vi "FPGA Main Default.vi"() -> ()   [LabVIEW 2016]
doc: "The myRIO v1.1 FPGA Shipping Personality. This personality contains support for:\n- 2 Analog Input Interrupt channel\n- 4 Digital Input Interrupt channel\n- 1 Timer\n- 1 Accelerometer\n- 1 Button\n- 4 LED\n- 10 Analog Input channels with 1 Sample\n- 6 Analog Output channels with 1 Sample\n- 40 Digital I/O channels with 1 Sample\n- 2 I2C channels\n- 4 Encoder channels\n- 6 PWM channels\n- 2 SPI channels"
uses:
  Sub VIs/Utilities/Start Boolean.ctl
  <vilib>/Platform/TimedLoop/XDataNode/timing_clust.ctl
  <vilib>/Platform/TimedLoop/XDataNode/nitl_modes.ctl
  <vilib>/Platform/TimedLoop/XDataNode/wakeup.ctl
  <vilib>/rvi/Emulation/niFpgaGetClockAttributes.vi
  <vilib>/rvi/Emulation/niFpgaSctlEmulationGetInTimedLoop.vi
  <vilib>/rvi/Emulation/niFpgaEmulationReportErrorSimple.vi
  <vilib>/rvi/eio/common/nirviEmuTemplateMethod_errors.vi
  <vilib>/rvi/Emulation/niFpgaCriticalErrorInLSC.vi
  <vilib>/rvi/Emulation/niFpgaProcessEmulError.vi
  <vilib>/rvi/Emulation/niFpgaEmulationIsFPGAContextNoSignature.vi
  <vilib>/rvi/errors/niFpgaSetErrorForExecOnDevCompSimple.vi
  <vilib>/rvi/eio/common/nirviEmuReportErrorAndStop.vi
  <vilib>/rvi/DataTransferAndStorage/Container/Common/niFpgaContainerGetUniqueNameForEmu.vi
  <vilib>/rvi/FIFO/Fifo_Resource/nirvififoEmulationSetSize.vi
  <vilib>/rvi/FIFO/Fifo_Resource/nirviFifoEmulationQueueMgr.vi
  <instcachedir>/0/nirviFifoEmulationQueueMgr_E5CAEC123FF24DC58D834DCA3CDAA9B5.lvgen/nirviFifoEmulationQueueMgr_E5CAEC123FF24DC58D834DCA3CDAA9B5_002.vi
  <vilib>/rvi/FIFO/Fifo_Resource/nirvififoEmulationDetermineInputValidOut.vi
  <vilib>/rvi/FIFO/Fifo_Resource/nirvififoEmulationCreateLock.vi
  <vilib>/rvi/FIFO/Fifo_Resource/nirvififoEmulationObtainLock.vi
  <vilib>/rvi/FIFO/Fifo_Resource/nirvififoEmulationReleaseLock.vi
  <vilib>/rvi/occurrence/nirviWaitOnOccurrenceBase.vi
  <vilib>/rvi/errors/nirviReportUnexpectedCaseInternalError.vi
  <vilib>/rvi/errors/nirviReportUnexpectedCaseInternalError (U32).vi
  <vilib>/Utility/error.llb/Clear Errors.vi
  <vilib>/rvi/DataTransferAndStorage/Container/Common/niFpgaContainerSetEmuInfo.vi
  <vilib>/eio/EIONode/EIONode.xnode
  <vilib>/rvi/DataTransferAndStorage/Container/XNode/niFpgaContainer.xnode
  <vilib>/rvi/FIFO/Fifo_Resource/nirvififoEmulationWrite.vi
  <vilib>/rvi/FIFO/Fifo_Resource/nirvififoEmulationRead.vi
  <vilib>/Platform/TimedLoop/XDataNode/XDataNode.xnode
  <vilib>/rvi/LocalResourceManager/LocalResourceManager.xnode
  <vilib>/Platform/TimedLoop/XDataNode/XDNodeRunTimeDep.lvlib
panel:
  in  "AO.A_0.VAL":u16
  in  "AO.A_1.VAL":u16
  in  "AO.B_0.VAL":u16
  in  "AO.B_1.VAL":u16
  out "AI.B_3.VAL":u16
  out "AI.B_2.VAL":u16
  out "AI.B_1.VAL":u16
  out "AI.B_0.VAL":u16
  out "AI.A_3.VAL":u16
  out "AI.A_2.VAL":u16
  out "AI.A_1.VAL":u16
  out "AI.A_0.VAL":u16
  out "DIO.B_7:0.IN":u8 format="%08b"
  in  "DIO.B_7:0.DIR":u8 format="%08b"
  in  "DIO.B_7:0.OUT":u8 format="%08b"
  in  "PWM.A_2.CS":u8=1
  in  "PWM.A_2.CNFG":u8=4
  out "PWM.A_2.CNTR":u16
  in  "PWM.A_2.MAX":u16=39999
  in  "PWM.A_2.CMP":u16=20000
  in  "PWM.A_1.CS":u8=1
  in  "PWM.A_1.CNFG":u8=4
  out "PWM.A_1.CNTR":u16
  in  "PWM.A_1.MAX":u16=39999
  in  "PWM.A_1.CMP":u16=20000
  in  "PWM.A_0.CS":u8=1
  in  "PWM.A_0.CNFG":u8=4
  out "PWM.A_0.CNTR":u16
  in  "PWM.A_0.CMP":u16=20000
  in  "PWM.A_0.MAX":u16=39999
  in  "SPI.A.DATO":u16
  out "SPI.A.DATI":u16
  in  "SPI.A.CNFG":u16=112
  in  "SPI.A.CNT":u16=19
  in  "SPI.B.CNT":u16=19
  in  "SPI.B.CNFG":u16=112 format="%0.0f"
  out "SPI.B.DATI":u16
  in  "SPI.B.DATO":u16
  in  "ENC.A.CNFG":u8 format="%08b"
  in  "ENC.B.CNFG":u8 format="%08b"
  out "ENC.A.CNTR":u32
  out "ENC.B.CNTR":u32
  out "ENC.A.STAT":u8 format="%08b"
  out "ENC.B.STAT":u8 format="%08b"
  in  "SPI.A.GO":T1
  out "SPI.A.STAT":u8 format="%08b"
  in  "SPI.B.GO":T1
  out "SPI.B.STAT":u8 format="%08b"
  out "I2C.B.STAT":u8 format="%08b"
  in  "I2C.B.CNTL":u8 format="%08b"
  out "I2C.A.STAT":u8 format="%08b"
  in  "I2C.A.CNTL":u8 format="%08b"
  in  "I2C.B.CNTR":u8=213
  in  "I2C.B.ADDR":u8 format="%08.0f"
  out "I2C.B.DATI":u8
  in  "I2C.B.DATO":u8
  in  "I2C.A.CNTR":u8=213
  in  "I2C.A.ADDR":u8 format="%08b"
  out "I2C.A.DATI":u8
  in  "I2C.A.DATO":u8
  in  "I2C.B.CNFG":u8=1 format="%08b"
  in  "I2C.A.CNFG":u8=1 format="%08b"
  in  "I2C.A.GO":T1
  in  "I2C.B.GO":T1
  out "SYS.AI.RDY":bool
  out "SYS.RDY":bool
  in  "PWM.B_2.CS":u8=1
  in  "PWM.B_2.CNFG":u8=4
  out "PWM.B_2.CNTR":u16
  in  "PWM.B_2.MAX":u16=39999
  in  "PWM.B_2.CMP":u16=20000
  in  "PWM.B_1.CS":u8=1
  in  "PWM.B_1.CNFG":u8=4
  out "PWM.B_1.CNTR":u16
  in  "PWM.B_1.MAX":u16=39999
  in  "PWM.B_1.CMP":u16=20000
  in  "PWM.B_0.CS":u8=1
  in  "PWM.B_0.CNFG":u8=4
  out "PWM.B_0.CNTR":u16
  in  "PWM.B_0.MAX":u16=39999
  in  "PWM.B_0.CMP":u16=20000
  out "DIO.A_7:0.IN":u8 format="%08b"
  in  "DIO.A_7:0.OUT":u8 format="%08b"
  in  "DIO.A_7:0.DIR":u8 format="%08b"
  out "AI.C_1.VAL":u16
  out "AI.C_0.VAL":u16
  in  "AO.C_0.VAL":u16
  in  "AO.C_1.VAL":u16
  in  "SYS.SELECTB":u8 format="%08b"
  in  "SYS.SELECTA":u8 format="%08b"
  out "DIO.A_15:8.IN":u8 format="%08b"
  in  "DIO.A_15:8.OUT":u8 format="%08b"
  in  "DIO.A_15:8.DIR":u8 format="%08b"
  out "DIO.B_15:8.IN":u8 format="%08b"
  in  "DIO.B_15:8.DIR":u8 format="%08b"
  in  "DIO.B_15:8.OUT":u8 format="%08b"
  out "AI.AudioIn_R.VAL":u16
  out "AI.AudioIn_L.VAL":u16
  in  "AO.AudioOut_R.VAL":u16
  in  "AO.AudioOut_L.VAL":u16
  in  "AO.SYS.GO":T1
  out "ACC.X.VAL":u16
  out "ACC.Y.VAL":u16
  out "SYS.ACC.RDY":bool
  out "ACC.Z.VAL":u16
  in  "DO.LED3:0":u8 format="%04b"
  out "DI.BTN":u8 format="%08b"
  out "AO.SYS.STAT":bool
  in  "IRQ.AI_A_3:0.CNFG":u8 format="%.0b"
  in  "IRQ.AI_A_0.THRESHOLD":u16
  in  "IRQ.AI_A_1.THRESHOLD":u16
  in  "IRQ.AI_A_0.NO":u8
  in  "IRQ.AI_A_1.NO":u8
  in  "IRQ.DIO_A_7:0.ENA":u8 format="%08b"
  in  "IRQ.DIO_A_7:0.RISE":u8 format="%08b"
  in  "IRQ.DIO_A_7:0.FALL":u8 format="%08b"
  in  "IRQ.DIO_A_0.NO":u8
  in  "IRQ.DIO_A_1.NO":u8
  in  "IRQ.DIO_A_2.NO":u8
  in  "IRQ.DIO_A_3.NO":u8
  in  "IRQ.DIO_A_3.CNT":u32
  in  "IRQ.DIO_A_2.CNT":u32
  in  "IRQ.DIO_A_1.CNT":u32
  in  "IRQ.DIO_A_0.CNT":u32
  in  "IRQ.AI_A_1.HYSTERESIS":u16=17
  in  "IRQ.TIMER.WRITE":u32
  in  "IRQ.TIMER.SETTIME":T1
  out "IRQ.TIMER.READ":u32
  in  "SPI.A.IRQ.NO":u8=15
  in  "SPI.B.IRQ.NO":u8=15
  in  "IRQ.AI_A_0.HYSTERESIS":u16=17
  in  "IRQ.DI_BTN.ENA":bool
  in  "IRQ.DI_BTN.RISE":bool
  in  "IRQ.DI_BTN.FALL":bool
  in  "IRQ.DI_BTN.CNT":u32
  in  "IRQ.DI_BTN.NO":u8
  # "System"
  # "Onboard Devices"
  # "Connector A"
  # "Connector B"
  # "Connector C"
  # "Audio Connector"
  # "Accelerometer"
  # "Analog Input"
  # "Analog Output"
  # "Digital I/O"
  # "PWM"
  # "SPI Master"
  # "Analog Input"
  # "Analog Output"
  # "Digital I/O"
  # "PWM"
  # "SPI Master"
  # "Analog Input"
  # "Analog Output"
  # "Digital I/O"
  # "Counters / PWM"
  # "Analog Input"
  # "Analog Output"
  # "IO Configuration"
  # "IO Configuration"
  # "IO Configuration"
  # "Encoders"
  # "Buttons & LEDs"
  # "Analog Interrupt"
  # "Digital Interrupt"
  # "Encoders"
  # "Encoders"
  # "Button Interrupt"
  # "I2C Master"
  # "I2C Master"
  # "Timer Interrupt"
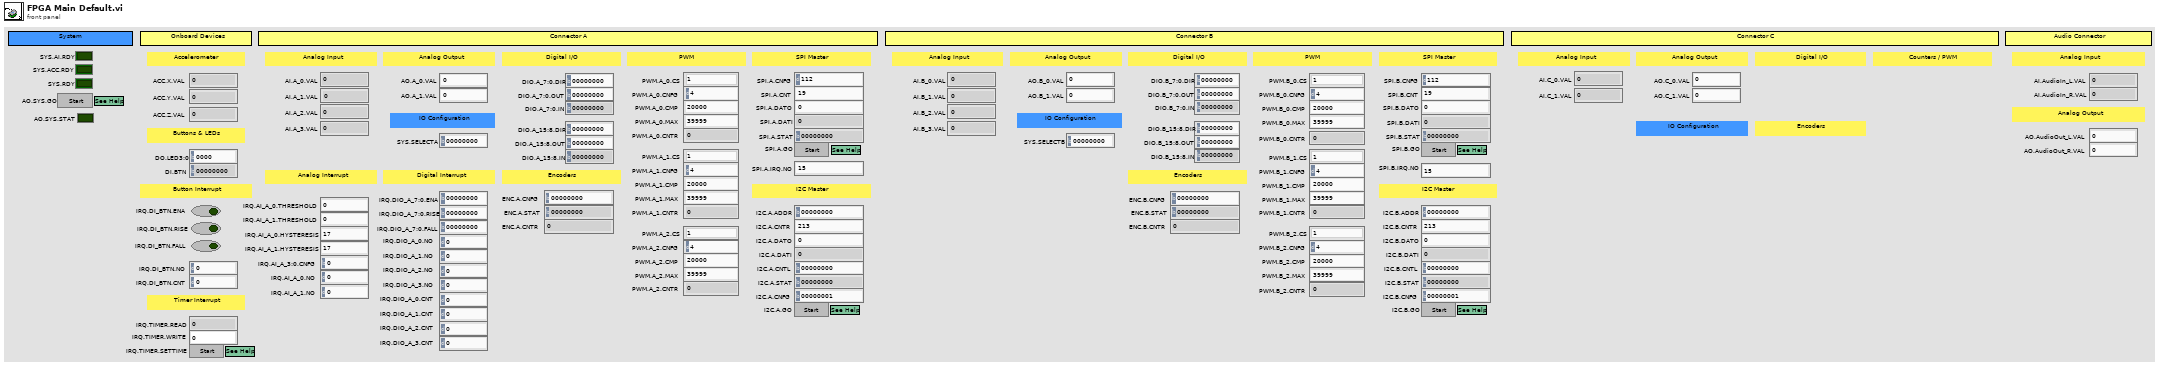
[diagram p1: front panel]
types:
  T1 = typedef "Start Boolean.ctl" = bool
  T2 = typedef "XDNodeRunTimeDep.lvlib/timing_clust.ctl" = cluster{"Expected End [f-1]":u64, "Actual End [f-1]":u64, "Finished Late? [f-1]":bool, "Expected End [i-1]":u64, "Actual End [i-1]":u64, "Finished Late? [i-1]":bool, "Expected Start [i]":u64, "Actual Start [i]":u64, "Expected Start [f]":u64, "Actual Start [f]":u64, "Source Name":string, "Structure Name":string, "Period":i64, "Deadline":i64, "Offset":i64, "Start":i64, "Priority":i32, "Timeout":i32, "Mode":T3, "Wakeup Reason":T4, "Error":errorcluster, "Source Type":string, "Secondary Source Type":string, "Global End Time":u64, "Global Start Time":u64, "Frame Duration":u64, "Iteration Duration":u64, "Assigned CPU":i32, "I/O Scan Engine Mode":u32}
  T3 = typedef "XDNodeRunTimeDep.lvlib/nitl_modes.ctl" = enum32{"No Change", "Process missed periods, maintain original phase", "Discard missed periods, maintain original phase", "Process missed periods, ignore original phase", "Discard missed periods, ignore original phase"}
  T4 = typedef "XDNodeRunTimeDep.lvlib/wakeup.ctl" = enum32{"Normal", "Aborted", "Asynchronous wakeup", "Timing source error", "Timed loop error", "Timeout"}
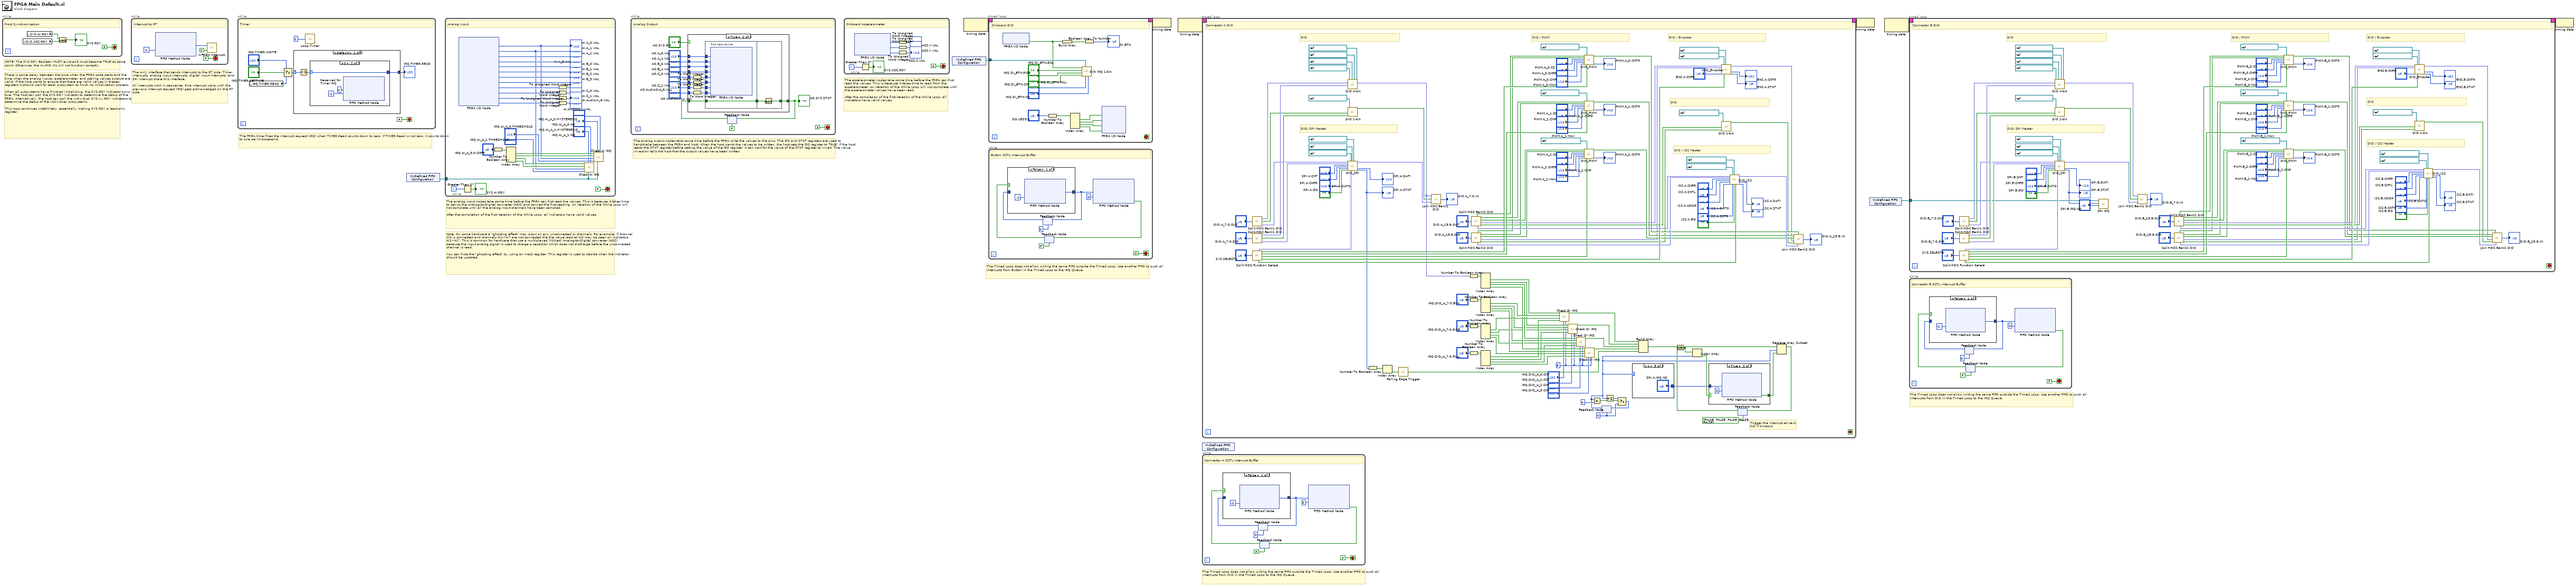
[diagram p0: block diagram]
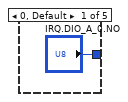
[diagram p9: hidden frame]
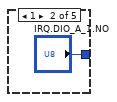
[diagram p10: hidden frame]
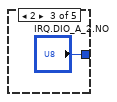
[diagram p11: hidden frame]
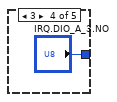
[diagram p12: hidden frame]
diagram:
  # "The Timed Loop does not allow writing the same FIFO outside the Timed Loop. Use another FIFO to push all interrupts from DIO in the Timed Loop to the IRQ Queue."
  # "The Timed Loop does not allow writing the same FIFO outside the Timed Loop. Use another FIFO to push all interrupts from Button in the Timed Loop to the IRQ Queue."
  # "The Timed Loop does not allow writing the same FIFO outside the Timed Loop. Use another FIFO to push all interrupts from DIO in the Timed Loop to the IRQ Queue."
  # "The accelerometer nodes take some time before the FPGA can first read the values. This is because it takes time to read from the accelerometer. An iteration of the While Loop will not complete until the accelerometer values have been read.\n\nAfter the completion of the first iteration of the While Loop, all indicators have valid values."
  # "The analog output nodes take some time before the FPGA write the values to the pins. The GO and STAT registers are used to handshake between the FPGA and host. When the host wants the values to be written, the host sets the GO register to TRUE. If the host reads the STAT register before setting the value of the GO register, it can wait for the value of the STAT register to invert. The value inversion tells the host that the output values have been written."
  # "The analog input nodes take some time before the FPGA can first read the values. This is because it takes time to set up the Analog-to-Digital converter (ADC) and convert the first reading. An iteration of the While Loop will not complete until all the analog input channels have been sampled.\n\nAfter the completion of the first iteration of the While Loop, all indicators have valid values."
  # "Note: On some hardware a \"ghosting effect\" may occur on any unconnected AI channels. For example, if channel AI0 is connected and channels AI1~AI7 are not connected the the value read at AI0 may be seen on indicators AI1~AI7. This is common for hardware that use a multiplexed (MUXed) Analog-to-Digital converter (ADC), because the input analog signal is used to charge a capacitor which does not discharge before the unconnected channel is read.\n\nYou can hide the \"ghosting effect\" by using an mask register. This register is used to decide when the indicator should be updated."
  # "The FPGA timer fires the interrupt request (IRQ) when TIMER.Read counts down to zero. If TIMER.Read is not zero, it counts down to one per microsecond."
  # "The only interface that sends interrupts to the RT side. Timer interrupts, analog input interrupts, digital input interrupts, and SPI interrupt share this interface.\n\nAll interrupts work in sequence. One interrupt waits until the previous interrupt request (IRQ) gets acknowledged on the RT side."
  # "NOTE: The SYS.RDY Boolean MUST exist and must become TRUE at some point. Otherwise, the myRIO VIs will not function correctly."
  # "There is some delay between the time when the FPGA code starts and the time when the analog inputs, accelerometer, and scaling values outputs are valid. If the host wants to ensure that there are valid values in theses registers it should wait for each subsystem to finish its initialization process. \n\nWhen all subsystems have finished initializinig, the SYS.RDY indicator turns true. The host can poll the SYS.RDY indicator to determine the status of the FPGA. Alternatively, the host can poll the individual SYS.xx.RDY indicators to determine the status of the individual subsystems.\n\nThis loop continues indefinitely, essentially making SYS.RDY a read-only register."
  n1 = while {
    stop <- FALSE stop-if-true
    # "Host Synchronization"
    n2 = local read "SYS.ACC.RDY"() -> (w11:bool)
    n3 = local read "SYS.AI.RDY"() -> (w13:bool)
    n4 = Compound Arithmetic op=AND(w13, w11) -> (→"SYS.RDY":bool)
  }
  n5 = while {
    stop <- FALSE stop-if-true
    # "Interrupt to RT"
    n6 = xnode ("FIFO Method Node")("Timeout"=-1) -> ("Element"=w16:u8)  [unwired: 1 in, 2 out]
    n7 = call <vilib>:"niFPGA Interrupt.vi"("Wait Until Cleared (F)"=TRUE, "IRQ Number (0)"=w16) -> ()  [unwired: 1 in]
  }
  n8 = while {
    stop <- FALSE stop-if-true
    # "Timer"
    n9 = local read "IRQ.TIMER.READ"() -> (w21:u32)
    n10 = Select(t="IRQ.TIMER.WRITE", s="IRQ.TIMER.SETTIME", f=w21) -> (s? t:f=w19:u32)
    n11 = case shown="Default" w19 {
      selector: w19 -> [w25 w28]
      tunnel: [w25 w26] -> w18
      frame 0 {
      }
      frame Default {
        n12 = Decrement(x=w28) -> (x-1=w27:u32)
        n13 = case shown="0" w27 {
          selector: w27 -> [w29 w32]
          tunnel: [w29 w32] -> w26
          frame Default {
          }
          frame 0 {
            w31 = u8 0  # Reserved for Timer IRQ
            n14 = xnode ("FIFO Method Node")("Element"=w31, "Timeout"=-1) -> ()  [unwired: 1 in, 2 out]
          }
        }
      }
    }
    "IRQ.TIMER.READ" <- w18
    n15 = call "Loop Timer"("Count(uSec)"=u8 1 ("Count(mSec)")) -> ()  [unwired: 1 out]
  }
  n16 = xnode "VI-Defined FIFO Configuration"() -> ("FIFO Out"=w3:refnum<k21>)
  n17 = while {
    tunnel: w3 -> [w34]
    i -> [w61]
    stop <- FALSE stop-if-true
    # "Analog Input"
    n18 = xnode "FPGA I/O Node"() -> ("ConnectorA/AI0"=w39:u16, "ConnectorA/AI1"=w38:u16, "ConnectorA/AI2"=→"AI.A_2.VAL":u16, "ConnectorA/AI3"=→"AI.A_3.VAL":u16, "ConnectorB/AI0"=→"AI.B_0.VAL":u16, "ConnectorB/AI1"=→"AI.B_1.VAL":u16, "ConnectorB/AI2"=→"AI.B_2.VAL":u16, "ConnectorB/AI3"=→"AI.B_3.VAL":u16, "ConnectorC/AI0"=w55:i16, "ConnectorC/AI1"=w54:i16, "AudioIn/Left"=w53:i16, "AudioIn/Right"=w52:i16)  [unwired: 12 in, 12 out]
    "AI.A_0.VAL" <- w39
    "AI.A_1.VAL" <- w38
    n19 = Greater Than 0?(x=w61) -> (x > 0?=→"SYS.AI.RDY":bool)
    n20 = Number To Boolean Array(number="IRQ.AI_A_3:0.CNFG") -> (Boolean array=w49:bool[])
    n21 = Index Array(array=w49) -> (element #1=w47:bool, element #2=w46:bool, element #3=w44:bool, element #4=w43:bool)  [unwired: 4 in]
    n22 = To Unsigned Word Integer(number=w55) -> (unsigned 16bit integer=→"AI.C_0.VAL":u16)
    n23 = To Unsigned Word Integer(number=w54) -> (unsigned 16bit integer=→"AI.C_1.VAL":u16)
    n24 = To Unsigned Word Integer(number=w53) -> (unsigned 16bit integer=→"AI.AudioIn_L.VAL":u16)
    n25 = To Unsigned Word Integer(number=w52) -> (unsigned 16bit integer=→"AI.AudioIn_R.VAL":u16)
    n26 = call "Check AI IRQ.vi"("Hysteresis"="IRQ.AI_A_1.HYSTERESIS", "FIFO In"=w34, "IRQ Number"="IRQ.AI_A_1.NO", "Threshold"="IRQ.AI_A_1.THRESHOLD", "Analog Value"=w38, "Rising Edge?"=w43, "Enable Interrupt?"=w44) -> ()  [unwired: 5 in]
    n27 = call "Check AI IRQ.vi"("Hysteresis"="IRQ.AI_A_0.HYSTERESIS", "FIFO In"=w34, "IRQ Number"="IRQ.AI_A_0.NO", "Threshold"="IRQ.AI_A_0.THRESHOLD", "Analog Value"=w39, "Rising Edge?"=w46, "Enable Interrupt?"=w47) -> ()  [unwired: 5 in]
  }
  n28 = while {
    stop <- FALSE stop-if-true
    # "Analog Output"
    n29 = feedback #1(FALSE) -> (w67:bool)
    n30 = case shown="True" "AO.SYS.GO" {
      tunnel: "AO.C_0.VAL" -> [_ w89]
      tunnel: "AO.C_1.VAL" -> [_ w88]
      tunnel: "AO.A_0.VAL" -> [_ w93]
      tunnel: "AO.A_1.VAL" -> [_ w92]
      tunnel: "AO.B_0.VAL" -> [_ w91]
      tunnel: "AO.B_1.VAL" -> [_ w90]
      tunnel: "AO.AudioOut_L.VAL" -> [_ w85]
      tunnel: "AO.AudioOut_R.VAL" -> [_ w84]
      tunnel: w67 -> [w78 w81]
      tunnel: [w78 w79] -> w65
      frame False {
      }
      frame True {
        n31 = To Word Integer(number=w89) -> (16bit integer=w87:i16)
        n32 = To Word Integer(number=w88) -> (16bit integer=w86:i16)
        n33 = To Word Integer(number=w85) -> (16bit integer=w83:i16)
        n34 = To Word Integer(number=w84) -> (16bit integer=w82:i16)
        n35 = flat-sequence {
          tunnel: w93 -> [w102]
          tunnel: w92 -> [w101]
          tunnel: w91 -> [w100]
          tunnel: w90 -> [w99]
          tunnel: w87 -> [w98]
          tunnel: w86 -> [w97]
          tunnel: w83 -> [w96]
          tunnel: w82 -> [w95]
          tunnel: w81 -> [w94]
          tunnel: [w94] -> w80
          tunnel: w80 -> [w104]
          tunnel: [w103] -> w79
          frame #0 {
            n36 = xnode "FPGA I/O Node"("ConnectorA/AO0"=w102, "ConnectorA/AO1"=w101, "ConnectorB/AO0"=w100, "ConnectorB/AO1"=w99, "ConnectorC/AO0"=w98, "ConnectorC/AO1"=w97, "AudioOut/Left"=w96, "AudioOut/Right"=w95) -> ()  [unwired: 8 in, 8 out]
          }
          frame #1 {
            n37 = Not(x=w104) -> (.not. x?=w103:bool)
          }
        }
      }
    }
    "AO.SYS.STAT" <- w65
    n38 = feedback-in #1(w65) -> ()
  }
  n39 = while {
    i -> [w109]
    stop <- FALSE stop-if-true
    # "Onboard Accelerometer"
    n40 = xnode "FPGA I/O Node"() -> ("AccelerationX"=w112:i16, "AccelerationY"=w111:i16, "AccelerationZ"=w110:i16)  [unwired: 3 in, 3 out]
    n41 = Greater Than 0?(x=w109) -> (x > 0?=→"SYS.ACC.RDY":bool)
    n42 = To Unsigned Word Integer(number=w112) -> (unsigned 16bit integer=→"ACC.X.VAL":u16)
    n43 = To Unsigned Word Integer(number=w111) -> (unsigned 16bit integer=→"ACC.Y.VAL":u16)
    n44 = To Unsigned Word Integer(number=w110) -> (unsigned 16bit integer=→"ACC.Z.VAL":u16)
  }
  n45 = xnode "VI-Defined FIFO Configuration"() -> ("FIFO Out"=w2:refnum<k21>)
  n46 = node-c288() -> (w5:T2)  [unwired: 1 in]
  n47 = timed-loop {
    timing: w5 -> [_]
    timing-out: [_] -> w4
    tunnel: w2 -> [w116]
    stop <- _ stop-if-true
    # "Onboard DIO"
    n48 = xnode "FPGA I/O Node"() -> ("Button0"=w120:bool)  [unwired: 1 in, 1 out]
    n49 = Number To Boolean Array(number="DO.LED3:0") -> (Boolean array=w125:bool[])
    n50 = Build Array(w120) -> (w128:bool[])
    n51 = Index Array(array=w125) -> (element #1=w124:bool, element #2=w123:bool, element #3=w122:bool, element #4=w121:bool)  [unwired: 4 in]
    n52 = call "DIO IRQ 1-bit.vi"("IRQ.NO"="IRQ.DI_BTN.NO", "IRQ.CNT"="IRQ.DI_BTN.CNT", "FIFO in"=w116, "IRQ.FALL"="IRQ.DI_BTN.FALL", "IRQ.RISE"="IRQ.DI_BTN.RISE", "IRQ.ENA"="IRQ.DI_BTN.ENA", "DIO"=w120) -> ()  [unwired: 5 in]
    n53 = Boolean Array To Number(Boolean array=w128) -> (number=→"DI.BTN":u8)
    n54 = xnode "FPGA I/O Node"("LED0"=w124, "LED1"=w123, "LED2"=w122, "LED3"=w121) -> ()  [unwired: 4 in, 4 out]
  }
  n55 = while {
    stop <- FALSE stop-if-true
    # "Button SCTL Interrupt Buffer"
    n56 = feedback #2(u8 0 ("Element")) -> (w133:u8)
    n57 = feedback #3(FALSE ("Timed Out?")) -> (w137:bool)
    n58 = case shown="False" w137 {
      tunnel: [w139 w141] -> w134
      tunnel: w133 -> [_ w141]
      frame False {
        n59 = xnode ("FIFO Method Node")("Timeout"=-1) -> ("Element"=w139:u8)  [unwired: 1 in, 2 out]
      }
      frame True {
      }
    }
    n60 = feedback-in #2(w134) -> ()
    n61 = xnode ("FIFO Method Node")("Element"=w134, "Timeout"=0) -> ("Timed Out?"=w135:bool)  [unwired: 1 in, 1 out]
    n62 = feedback-in #3(w135) -> ()
  }
  n63 = node-c288(w4) -> ()
  n64 = node-c288() -> (w9:T2)  [unwired: 1 in]
  n65 = xnode "VI-Defined FIFO Configuration"() -> ()  [unwired: 1 out]
  n66 = while {
    stop <- FALSE stop-if-true
    # "Connector A SCTL Interrupt Buffer"
    n67 = feedback #4(u8 0 ("Element")) -> (w144:u8)
    n68 = feedback #5(FALSE ("Timed Out?")) -> (w148:bool)
    n69 = case shown="False" w148 {
      tunnel: [w150 w152] -> w145
      tunnel: w144 -> [_ w152]
      frame False {
        n70 = xnode ("FIFO Method Node")("Timeout"=-1) -> ("Element"=w150:u8)  [unwired: 1 in, 2 out]
      }
      frame True {
      }
    }
    n71 = feedback-in #4(w145) -> ()
    n72 = xnode ("FIFO Method Node")("Element"=w145, "Timeout"=0) -> ("Timed Out?"=w146:bool)  [unwired: 1 in, 1 out]
    n73 = feedback-in #5(w146) -> ()
  }
  n74 = timed-loop {
    timing: w9 -> [_]
    timing-out: [_] -> w8
    stop <- _ stop-if-true
    w153 = u16 5 ("Debounce Ticks")
    w154 = u8 0
    # "Trigger the interrupt at next \ntick if timeout"
    # "DIO / Encoder"
    # "DIO / I2C Master"
    # "DIO / PWM"
    # "DIO"
    # "DIO"
    # "DIO/ SPI Master"
    # "Connector A DIO"
    n75 = call "Split HDC Bank1 DIO.vi"("IN 7:0"="DIO.A_7:0.OUT") -> ("OUT 3:0"=w289:fxp<+,4,4>, "OUT 4"=w208:bool, "OUT 7:5"=w286:fxp<+,3,3>)
    n76 = call "Split HDC Bank1 DIO.vi"("IN 7:0"="DIO.A_7:0.DIR") -> ("OUT 3:0"=w288:fxp<+,4,4>, "OUT 4"=w287:bool, "OUT 7:5"=w285:fxp<+,3,3>)
    n77 = call "Split HDC Function Select.vi"("IN 7:0"="SYS.SELECTA") -> ("OUT 1:0"=w228:fxp<+,2,2>, "OUT 7"=w223:bool, "OUT 2"=w227:bool, "OUT 3"=w226:bool, "OUT 4"=w225:bool, "OUT 5"=w224:bool)
    n78 = call "DIO 4-bit.vi"("DIO0 Refnum"=refnum<k21> "ConnectorA/DIO0", "DIO1 Refnum"=refnum<k21> "ConnectorA/DIO1", "DIO2 Refnum"=refnum<k21> "ConnectorA/DIO2", "DIR 3:0"=w288, "OUT 3:0"=w289, "DIO3 Refnum"=refnum<k21> "ConnectorA/DIO3") -> ("IN 3:0"=w176:fxp<+,4,4>)  [unwired: 5 in]
    n79 = call "DIO 1-bit.vi"("DIR"=w287, "OUT"=w208, "DIO Refnum"=refnum<k21> "ConnectorA/DIO4") -> ("IN"=w175:bool)  [unwired: 8 in]
    n80 = call "DIO_SPI.vi"("DIO.2:0.OUT"=w286, "DIO.2:0.DIR"=w285, "SPI.CNT"="SPI.A.CNT", "SPI.CNFG"="SPI.A.CNFG", "SPI.DATO"="SPI.A.DATO", "SPI.GO"="SPI.A.GO", "DIO.2/SPI.MOSI Refnum"=refnum<k21> "ConnectorA/DIO7" ("DIO.2/SPI.SCLK"), "SELECT.1:0"=w228, "DIO.1/SPI.MISO Refnum"=refnum<k21> "ConnectorA/DIO6" ("DIO.1/SPI.MOSI"), "DIO.0/SPI.SCLK Refnum"=refnum<k21> "ConnectorA/DIO5" ("DIO.0/SPI.MISO")) -> ("DIO.2:0.IN"=w261:fxp<+,3,3>, "SPI.DATI"=→"SPI.A.DATI":u16, "SPI.STAT"=w161:u8)  [unwired: 7 in]
    "SPI.A.STAT" <- w161
    n81 = Number To Boolean Array(number=w161) -> (Boolean array=w163:bool[])
    n82 = Index Array(array=w163) -> (element=w162:bool)  [unwired: 1 in]
    n83 = call "Falling Edge Trigger.vi"("Signal"=w162) -> ("Trigger?"=w160:bool)
    n84 = call "Join HDC Bank1 DIO.vi"("IN 7:5"=w261, "IN 4"=w175, "IN 3:0"=w176) -> ("OUT 7:0"=→"DIO.A_7:0.IN":u8)
    n85 = Number To Boolean Array(number=w176) -> (Boolean array=w201:bool[])
    n86 = Number To Boolean Array(number="IRQ.DIO_A_7:0.ENA") -> (Boolean array=w207:bool[])
    n87 = Number To Boolean Array(number="IRQ.DIO_A_7:0.RISE") -> (Boolean array=w206:bool[])
    n88 = Number To Boolean Array(number="IRQ.DIO_A_7:0.FALL") -> (Boolean array=w205:bool[])
    n89 = call "Split HDC Bank2 DIO.vi"("IN 7:0"="DIO.A_15:8.OUT") -> ("OUT 5"=w210:bool, "OUT 7:6"=w232:fxp<+,2,2>, "OUT 4:3"=w212:fxp<+,2,2>, "OUT 2"=w214:bool, "OUT 0"=w218:bool, "OUT 1"=w217:bool)  [unwired: 2 in]
    n90 = call "Split HDC Bank2 DIO.vi"("IN 7:0"="DIO.A_15:8.DIR") -> ("OUT 5"=w209:bool, "OUT 7:6"=w231:fxp<+,2,2>, "OUT 4:3"=w211:fxp<+,2,2>, "OUT 2"=w213:bool, "OUT 0"=w216:bool, "OUT 1"=w215:bool)  [unwired: 2 in]
    n91 = Index Array(array=w201) -> (element #1=w182:bool, element #2=w197:bool, element #3=w196:bool, element #4=w195:bool)  [unwired: 4 in]
    n92 = Index Array(array=w207) -> (element #1=w200:bool, element #2=w194:bool, element #3=w193:bool, element #4=w192:bool)  [unwired: 4 in]
    n93 = Index Array(array=w206) -> (element #1=w199:bool, element #2=w191:bool, element #3=w190:bool, element #4=w189:bool)  [unwired: 4 in]
    n94 = Index Array(array=w205) -> (element #1=w198:bool, element #2=w188:bool, element #3=w187:bool, element #4=w186:bool)  [unwired: 4 in]
    n95 = call "Check DI IRQ.vi"("Debounce Ticks"=w153, "Count"="IRQ.DIO_A_0.CNT", "On Falling Edge?"=w198, "On Rising Edge?"=w199, "Enable Interrupt?"=w200, "Digital In"=w182) -> ("Trigger?"=w173:bool)  [unwired: 5 in]
    n96 = call "Check DI IRQ.vi"("Debounce Ticks"=w153, "Count"="IRQ.DIO_A_1.CNT", "On Falling Edge?"=w188, "On Rising Edge?"=w191, "Enable Interrupt?"=w194, "Digital In"=w197) -> ("Trigger?"=w172:bool)  [unwired: 5 in]
    n97 = call "Check DI IRQ.vi"("Debounce Ticks"=w153, "Count"="IRQ.DIO_A_2.CNT", "On Falling Edge?"=w187, "On Rising Edge?"=w190, "Enable Interrupt?"=w193, "Digital In"=w196) -> ("Trigger?"=w171:bool)  [unwired: 5 in]
    n98 = call "DIO_PWM.vi"("DIO.OUT"=w218, "DIO.DIR"=w216, "PWM.CS"="PWM.A_0.CS", "PWM.CNFG"="PWM.A_0.CNFG", "PWM.CMP"="PWM.A_0.CMP", "PWM.MAX"="PWM.A_0.MAX", "DIO/PWM"=refnum<k21> "ConnectorA/DIO8", "SELECT"=w227) -> ("DIO.IN"=w222:bool, "PWM.CNTR"=→"PWM.A_0.CNTR":u16)  [unwired: 10 in]
    n99 = call "DIO_PWM.vi"("DIO.OUT"=w217, "DIO.DIR"=w215, "PWM.CS"="PWM.A_1.CS", "PWM.CNFG"="PWM.A_1.CNFG", "PWM.CMP"="PWM.A_1.CMP", "PWM.MAX"="PWM.A_1.MAX", "DIO/PWM"=refnum<k21> "ConnectorA/DIO9", "SELECT"=w226) -> ("DIO.IN"=w221:bool, "PWM.CNTR"=→"PWM.A_1.CNTR":u16)  [unwired: 10 in]
    n100 = call "DIO_PWM.vi"("DIO.OUT"=w214, "DIO.DIR"=w213, "PWM.CS"="PWM.A_2.CS", "PWM.CNFG"="PWM.A_2.CNFG", "PWM.CMP"="PWM.A_2.CMP", "PWM.MAX"="PWM.A_2.MAX", "DIO/PWM"=refnum<k21> "ConnectorA/DIO10", "SELECT"=w225) -> ("DIO.IN"=w220:bool, "PWM.CNTR"=→"PWM.A_2.CNTR":u16)  [unwired: 10 in]
    n101 = call "Check DI IRQ.vi"("Debounce Ticks"=w153, "Count"="IRQ.DIO_A_3.CNT", "On Falling Edge?"=w186, "On Rising Edge?"=w189, "Enable Interrupt?"=w192, "Digital In"=w195) -> ("Trigger?"=w170:bool)  [unwired: 5 in]
    n102 = feedback #6(w154) -> (w156:u8)
    n103 = Less?(x=w156, y=4 ("x")) -> (x < y?=w158:bool)
    n104 = Increment(x=w156) -> (x+1=w157:u8)
    n105 = Select(t=w157, s=w158, f=w154) -> (s? t:f=w155:u8)
    n106 = feedback-in #6(w155) -> ()
    n107 = case shown="4" w156 {
      tunnel: ["IRQ.DIO_A_0.NO" "IRQ.DIO_A_1.NO" "IRQ.DIO_A_2.NO" "IRQ.DIO_A_3.NO" "SPI.A.IRQ.NO"] -> w185
      frame 0, Default {
      }
      frame 1 {
      }
      frame 2 {
      }
      frame 3 {
      }
      frame 4 {
      }
    }
    n108 = Build Array(w173, w172, w171, w170, w160) -> (w168:bool[])
    n109 = call "DIO_Encoder.vi"("DIO.1:0.OUT"=w212, "DIO.1:0.DIR"=w211, "QE.CNFG"="ENC.A.CNFG", "DIO.1/QE.B"=refnum<k21> "ConnectorA/DIO12", "SELECT"=w224, "DIO.0/QE.A"=refnum<k21> "ConnectorA/DIO11") -> ("DIO.1:0.IN"=w219:fxp<+,2,2>, "QE.CNTR"=→"ENC.A.CNTR":u32, "QE.STAT"=→"ENC.A.STAT":u8)  [unwired: 11 in]
    n110 = call "DIO 1-bit.vi"("DIR"=w209, "OUT"=w210, "DIO Refnum"=refnum<k21> "ConnectorA/DIO13") -> ("IN"=w174:bool)  [unwired: 8 in]
    n111 = call "DIO_I2C.vi"("DIO.1:0.OUT"=w232, "DIO.1:0.DIR"=w231, "I2C.CNFG"="I2C.A.CNFG", "I2C.CNTL"="I2C.A.CNTL", "I2C.ADDR"="I2C.A.ADDR", "I2C.DATO"="I2C.A.DATO", "DIO.1/I2C.SDA"=refnum<k21> "ConnectorA/DIO15" ("DIO.1/I2C.SCL"), "I2C.CNTR"="I2C.A.CNTR", "DIO.0/I2C.SCL"=refnum<k21> "ConnectorA/DIO14" ("DIO.0/I2C.SDA"), "Execute?"="I2C.A.GO", "SELECT"=w223) -> ("DIO.1:0.IN"=w230:fxp<+,2,2>, "I2C.DATI"=→"I2C.A.DATI":u8, "I2C.STAT"=→"I2C.A.STAT":u8)  [unwired: 6 in]
    n112 = feedback #7(bool[] [FALSE, FALSE, FALSE, FALSE, FALSE] ("initialized array")) -> (w164:bool[])
    n113 = Or(x=w168, y=w164) -> (x .or. y?=w169:bool[])
    n114 = Index Array(array=w169, index=w156) -> (element=w167:bool)
    n115 = case shown="True" w167 {
      selector: w167 -> [w290 _]
      tunnel: [w290 w291] -> w166
      tunnel: w185 -> [_ w292]
      frame False {
      }
      frame True {
        n116 = xnode ("FIFO Method Node")("Element"=w292, "Timeout"=0) -> ("Timed Out?"=w291:bool)  [unwired: 1 in, 1 out]
      }
    }
    n117 = Replace Array Subset(array=w169, new element=w166, index=w156) -> (w165:bool[])
    n118 = feedback-in #7(w165) -> ()
    n119 = call "Join HDC Bank2 DIO.vi"("IN 7:6"=w230, "IN 5"=w174, "IN 4:3"=w219, "IN 0"=w222, "IN 2"=w220, "IN 1"=w221) -> ("OUT 7:0"=→"DIO.A_15:8.IN":u8)  [unwired: 4 in]
  }
  n120 = node-c288(w8) -> ()
  n121 = xnode "VI-Defined FIFO Configuration"() -> ("FIFO Out"=w1:refnum<k21>)
  n122 = node-c288() -> (w7:T2)  [unwired: 1 in]
  n123 = timed-loop {
    timing: w7 -> [_]
    timing-out: [_] -> w6
    tunnel: w1 -> [w301]
    stop <- _ stop-if-true
    # "DIO / Encoder"
    # "DIO / I2C Master"
    # "DIO / PWM"
    # "DIO"
    # "DIO"
    # "DIO/ SPI Master"
    # "Connector B DIO"
    n124 = call "Split HDC Bank1 DIO.vi"("IN 7:0"="DIO.B_7:0.OUT") -> ("OUT 3:0"=w390:fxp<+,4,4>, "OUT 4"=w388:bool, "OUT 7:5"=w386:fxp<+,3,3>)
    n125 = call "Split HDC Bank1 DIO.vi"("IN 7:0"="DIO.B_7:0.DIR") -> ("OUT 3:0"=w389:fxp<+,4,4>, "OUT 4"=w387:bool, "OUT 7:5"=w385:fxp<+,3,3>)
    n126 = call "Split HDC Function Select.vi"("IN 7:0"="SYS.SELECTB") -> ("OUT 1:0"=w362:fxp<+,2,2>, "OUT 7"=w357:bool, "OUT 2"=w361:bool, "OUT 3"=w360:bool, "OUT 4"=w359:bool, "OUT 5"=w358:bool)
    n127 = call "DIO 4-bit.vi"("DIO0 Refnum"=refnum<k21> "ConnectorB/DIO0", "DIO1 Refnum"=refnum<k21> "ConnectorB/DIO1", "DIO2 Refnum"=refnum<k21> "ConnectorB/DIO2", "DIR 3:0"=w389, "OUT 3:0"=w390, "DIO3 Refnum"=refnum<k21> "ConnectorB/DIO3") -> ("IN 3:0"=w368:fxp<+,4,4>)  [unwired: 5 in]
    n128 = call "DIO 1-bit.vi"("DIR"=w387, "OUT"=w388, "DIO Refnum"=refnum<k21> "ConnectorB/DIO4") -> ("IN"=w367:bool)  [unwired: 8 in]
    n129 = call "DIO_SPI.vi"("DIO.2:0.OUT"=w386, "DIO.2:0.DIR"=w385, "SPI.CNT"="SPI.B.CNT", "SPI.CNFG"="SPI.B.CNFG", "SPI.DATO"="SPI.B.DATO", "SPI.GO"="SPI.B.GO", "DIO.2/SPI.MOSI Refnum"=refnum<k21> "ConnectorB/DIO7" ("DIO.2/SPI.SCLK"), "SELECT.1:0"=w362, "DIO.1/SPI.MISO Refnum"=refnum<k21> "ConnectorB/DIO6" ("DIO.1/SPI.MOSI"), "DIO.0/SPI.SCLK Refnum"=refnum<k21> "ConnectorB/DIO5" ("DIO.0/SPI.MISO")) -> ("DIO.2:0.IN"=w366:fxp<+,3,3>, "SPI.DATI"=→"SPI.B.DATI":u16, "SPI.STAT"=w302:u8)  [unwired: 7 in]
    "SPI.B.STAT" <- w302
    n130 = call "SPI IRQ.vi"("SPI.A.IRQ.NO"="SPI.B.IRQ.NO", "SPI.STAT"=w302, "FIFO In"=w301) -> ()  [unwired: 9 in]
    n131 = call "Join HDC Bank1 DIO.vi"("IN 7:5"=w366, "IN 4"=w367, "IN 3:0"=w368) -> ("OUT 7:0"=→"DIO.B_7:0.IN":u8)
    n132 = call "Split HDC Bank2 DIO.vi"("IN 7:0"="DIO.B_15:8.OUT") -> ("OUT 5"=w314:bool, "OUT 7:6"=w365:fxp<+,2,2>, "OUT 4:3"=w315:fxp<+,2,2>, "OUT 2"=w316:bool, "OUT 0"=w318:bool, "OUT 1"=w317:bool)  [unwired: 2 in]
    n133 = call "Split HDC Bank2 DIO.vi"("IN 7:0"="DIO.B_15:8.DIR") -> ("OUT 5"=w309:bool, "OUT 7:6"=w364:fxp<+,2,2>, "OUT 4:3"=w310:fxp<+,2,2>, "OUT 2"=w311:bool, "OUT 0"=w313:bool, "OUT 1"=w312:bool)  [unwired: 2 in]
    n134 = call "DIO_PWM.vi"("DIO.OUT"=w318, "DIO.DIR"=w313, "PWM.CS"="PWM.B_0.CS", "PWM.CNFG"="PWM.B_0.CNFG", "PWM.CMP"="PWM.B_0.CMP", "PWM.MAX"="PWM.B_0.MAX", "DIO/PWM"=refnum<k21> "ConnectorB/DIO8", "SELECT"=w361) -> ("DIO.IN"=w308:bool, "PWM.CNTR"=→"PWM.B_0.CNTR":u16)  [unwired: 10 in]
    n135 = call "DIO_PWM.vi"("DIO.OUT"=w317, "DIO.DIR"=w312, "PWM.CS"="PWM.B_1.CS", "PWM.CNFG"="PWM.B_1.CNFG", "PWM.CMP"="PWM.B_1.CMP", "PWM.MAX"="PWM.B_1.MAX", "DIO/PWM"=refnum<k21> "ConnectorB/DIO9", "SELECT"=w360) -> ("DIO.IN"=w307:bool, "PWM.CNTR"=→"PWM.B_1.CNTR":u16)  [unwired: 10 in]
    n136 = call "DIO_PWM.vi"("DIO.OUT"=w316, "DIO.DIR"=w311, "PWM.CS"="PWM.B_2.CS", "PWM.CNFG"="PWM.B_2.CNFG", "PWM.CMP"="PWM.B_2.CMP", "PWM.MAX"="PWM.B_2.MAX", "DIO/PWM"=refnum<k21> "ConnectorB/DIO10", "SELECT"=w359) -> ("DIO.IN"=w306:bool, "PWM.CNTR"=→"PWM.B_2.CNTR":u16)  [unwired: 10 in]
    n137 = call "DIO_Encoder.vi"("DIO.1:0.OUT"=w315, "DIO.1:0.DIR"=w310, "QE.CNFG"="ENC.B.CNFG", "DIO.1/QE.B"=refnum<k21> "ConnectorB/DIO12", "SELECT"=w358, "DIO.0/QE.A"=refnum<k21> "ConnectorB/DIO11") -> ("DIO.1:0.IN"=w305:fxp<+,2,2>, "QE.CNTR"=→"ENC.B.CNTR":u32, "QE.STAT"=→"ENC.B.STAT":u8)  [unwired: 11 in]
    n138 = call "DIO 1-bit.vi"("DIR"=w309, "OUT"=w314, "DIO Refnum"=refnum<k21> "ConnectorB/DIO13") -> ("IN"=w304:bool)  [unwired: 8 in]
    n139 = call "DIO_I2C.vi"("DIO.1:0.OUT"=w365, "DIO.1:0.DIR"=w364, "I2C.CNFG"="I2C.B.CNFG", "I2C.CNTL"="I2C.B.CNTL", "I2C.ADDR"="I2C.B.ADDR", "I2C.DATO"="I2C.B.DATO", "DIO.1/I2C.SDA"=refnum<k21> "ConnectorB/DIO15" ("DIO.1/I2C.SCL"), "I2C.CNTR"="I2C.B.CNTR", "DIO.0/I2C.SCL"=refnum<k21> "ConnectorB/DIO14" ("DIO.0/I2C.SDA"), "Execute?"="I2C.B.GO", "SELECT"=w357) -> ("DIO.1:0.IN"=w363:fxp<+,2,2>, "I2C.DATI"=→"I2C.B.DATI":u8, "I2C.STAT"=→"I2C.B.STAT":u8)  [unwired: 6 in]
    n140 = call "Join HDC Bank2 DIO.vi"("IN 7:6"=w363, "IN 5"=w304, "IN 4:3"=w305, "IN 0"=w308, "IN 2"=w306, "IN 1"=w307) -> ("OUT 7:0"=→"DIO.B_15:8.IN":u8)  [unwired: 4 in]
  }
  n141 = while {
    stop <- FALSE stop-if-true
    # "Connector B SCTL Interrupt Buffer"
    n142 = feedback #8(u8 0 ("Element")) -> (w395:u8)
    n143 = feedback #9(FALSE ("Timed Out?")) -> (w399:bool)
    n144 = case shown="False" w399 {
      tunnel: [w401 w403] -> w396
      tunnel: w395 -> [_ w403]
      frame False {
        n145 = xnode ("FIFO Method Node")("Timeout"=-1) -> ("Element"=w401:u8)  [unwired: 1 in, 2 out]
      }
      frame True {
      }
    }
    n146 = feedback-in #8(w396) -> ()
    n147 = xnode ("FIFO Method Node")("Element"=w396, "Timeout"=0) -> ("Timed Out?"=w397:bool)  [unwired: 1 in, 1 out]
    n148 = feedback-in #9(w397) -> ()
  }
  n149 = node-c288(w6) -> ()
